vi "SVT UFF58 Write Spectrum (Complex) (N Ch).vi"(0 "file refnum":refnum<k20>, 1 "ID lines (1-3)":T8[](array[typedef]), 2 "data precision (double-precision:1)":T1=1 items=["single-precision", "double-precision"], 5 "real part":cluster{"x0":dbl, "dx":dbl, "Y Real":dbl[]}[](array[cluster]) {"Y Real" format="%.2f"; "dx" format="%.2f"; "x0" format="%.2f"}, 7 "imaginary part":cluster{"x0":dbl, "dx":dbl, "Y Im":dbl[]}[](array[cluster]) {"Y Im" format="%.2f"; "dx" format="%.2f"; "x0" format="%.2f"}, 9 "spectrum info":T2[](array[typedef]) {"x-axis units" items=["Time (s)"=0, "Frequency-CB (Hz)"=1, "Frequency-CPB (Hz)"=1248, "Frequency-Arbitrary (Hz)"=2357, "Quefrency (s)"=2, "Revolutions (rev)"=3, "Order"=4, "Speed (RPM)"=11, "Speed (rad/s)"=21, "Index"=65535]; "weighting filter" items=["Linear", "A-weighting", "B-weighting", "C-weighting", "ITU-R 468-4", "Dolby", "CCITT", "C-message", "Wb", "Wc", "Wd", "We", "Wf", "Wh", "Wj", "Wk", "Wm", "AES17 20 kHz lowpass", "AES17 40 kHz lowpass", "AES17 20 kHz highpass", "AES17 40 kHz highpass"]; "dB reference [EU]" format="%.2f"; "engineering units" items=["custom..."=0, "V"=1, "A"=21, "C"=30, "pC"=31, "s"=32, "-"=29, "Pa"=2, "N"=20, "g"=3, "m/s^2"=4, "m/s"=5, "m"=6, "mm/s"=12, "mm"=13, "micron/s"=14, "micron"=15, "in/s^2"=7, "in/s"=8, "in"=9, "mil/s"=10, "mil"=11, "rad/s^2"=16, "rad/s"=17, "rad"=18, "deg/s^2"=26, "deg/s"=27, "deg"=28, "RPM"=22, "cycle/s^2"=23, "Hz"=24, "cycle"=25, "strain"=19]; "spectral info"."window" items=["None "=0, "Hanning"=1, "Hamming"=2, "Blackman-Harris"=3, "Exact Blackman"=4, "Blackman"=5, "Flat Top"=6, "4 Term B-Harris "=7, "7 Term B-Harris"=8, "Low Sidelobe"=9, "Force - Exponential"=10, "Gaussian"=62]}, 11 "error in (no error)":errorcluster) -> (4 "dup file refnum":refnum<k20>, 6 "function refnums":refnum<k20>[](array[refnum]), 15 "error out":errorcluster)   [LabVIEW 2017, in "SoundVib_UFF58.lvlib"]
doc: "Writes data to the UFF58 (universal file format) file specified by the <B>file refnum</B> input. This VI also writes the fields in records 1, 2, and 3, <B>ID lines (1-3)</B>. You can write a single time domain waveform, multiple time domain waveforms, a single real frequency spectrum, multiple real frequency spectra, a single complex frequency spectrum, multiple complex frequency spectra, or generic data to a UFF file. If a frequency spectrum is in decibels, this VI converts the spectrum to linear before writing to the UFF58 file. The default instance, SVT UFF58 Write Time Waveform (1 Ch), writes a single time domain waveform to the file specified by the <B>file refnum</B> input. Wire data to the <B>file refnum</B> input to determine the polymorphic instance to use or manually select the instance."
uses:
  <vilib>/addons/Sound and Vibration/svt_UFF58/SoundVib_UFF58.lvlib
  <vilib>/addons/Sound and Vibration/svt_UFF58/subVIs/sv_IDLines123.ctl
  <vilib>/addons/_NISVFA/_Shared subVIs/Controls/svc_Spectrum Info.ctl
  <vilib>/addons/_NISVFA/_Shared subVIs/Controls/svc_X-Axis Units.ctl
  <vilib>/addons/_NISVFA/_Shared subVIs/Controls/svc_Spectrum Type.ctl
  <vilib>/addons/_NISVFA/_Shared subVIs/Controls/svc_Engineering Units Text Ring.ctl
  <vilib>/addons/_NISVFA/_Shared subVIs/Controls/svc_Weighting Filter Text Ring.ctl
  <vilib>/addons/_NISVFA/_Shared subVIs/Controls/svc_Complimentary Spectrum Units.ctl
  <vilib>/addons/Sound and Vibration/svt_UFF58/subVIs/sv_UFF58 Data Precision.ctl
  <vilib>/addons/Sound and Vibration/svt_UFF58/subVIs/sv_UFF58 Check Data Valid (Freq - Complex) (N Ch).vi
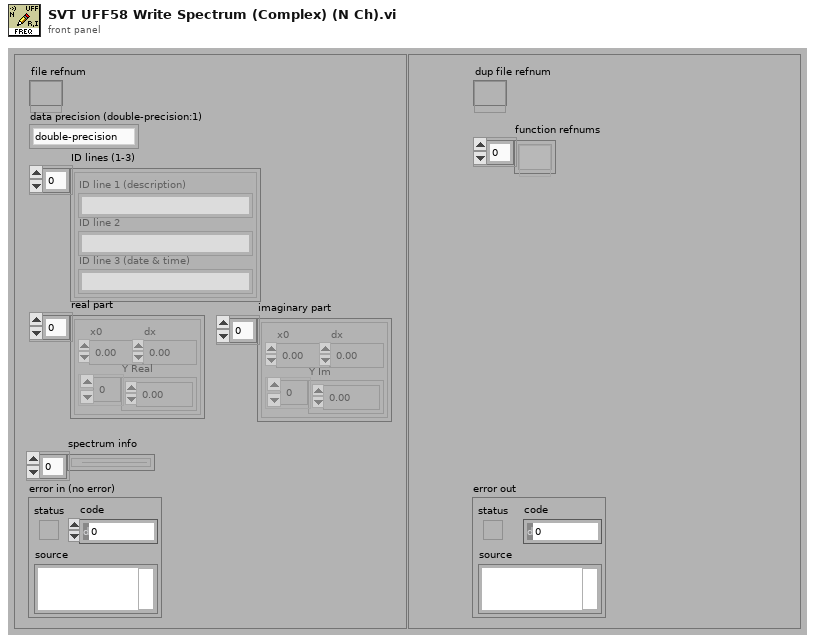
[diagram p1: front panel]
types:
  T1 = typedef "SoundVib_UFF58.lvlib/sv_UFF58 Data Precision.ctl" = u32
  T2 = typedef "svc_Spectrum Info.ctl" = cluster{"channel name":string, "description":string, "x-axis units":T3, "spectral info":cluster{"spectrum type":T4, "linear/dB":enum16{"linear", "dB"}, "window":u16, "window size":i32, "FFT size":i32}, "engineering units":T5, "custom label":string, "dB reference [EU]":dbl, "peak units":enum16{"rms", "peak", "peak-peak"}, "weighting filter":T6, "spectral density?":bool, "unit label":string, "spectrum skewed?":bool, "complimentary spectrum units":T7}
  T3 = typedef "svc_X-Axis Units.ctl" = u16
  T4 = typedef "svc_Spectrum Type.ctl" = enum16{"FFT Spectrum [complex]", "Amplitude [Magnitude]", "Power [Magnitude^2]", "Cross Spectrum [complex]", "Frequency Response [Complex]"}
  T5 = typedef "svc_Engineering Units Text Ring.ctl" = u16
  T6 = typedef "svc_Weighting Filter Text Ring.ctl" = u16
  T7 = typedef "svc_Complimentary Spectrum Units.ctl" = enum16{"none", "radians", "degrees", "cycles", "imaginary"}
  T8 = typedef "SoundVib_UFF58.lvlib/sv_IDLines123.ctl" = cluster{"ID line 1 (description)":string, "ID line 2":string, "ID line 3 (date & time)":string}
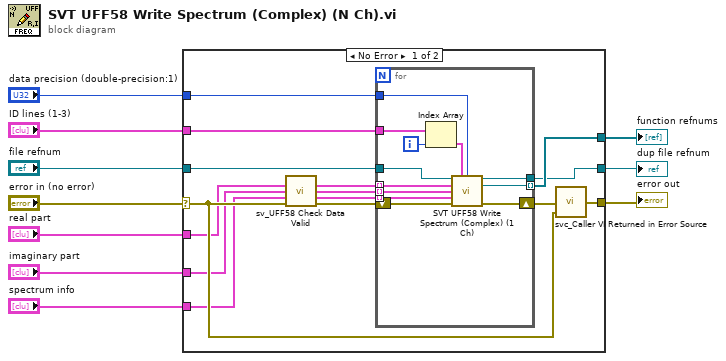
[diagram p0: block diagram]
diagram:
  n1 = case shown="No Error" "error in (no error)" {
    selector: "error in (no error)" -> [w17 w39]
    tunnel: "file refnum" -> [w25 w38]
    tunnel: "spectrum info" -> [w12 _]
    tunnel: "ID lines (1-3)" -> [w14 _]
    tunnel: [w24 _] -> w7
    tunnel: "real part" -> [w16 _]
    tunnel: "imaginary part" -> [w15 _]
    tunnel: [w18 w39] -> w4
    tunnel: [w23 w38] -> w3
    tunnel: "data precision (double-precision:1)" -> [w13 _]
    frame No Error {
      n2 = call-poly <vilib>:"sv_UFF58 Check Data Valid.vi"("real part in"=w16, "imaginary part in"=w15, "spectrum info in"=w12, "error in (no error)"=w17) -> ("real part out"=w21:cluster{"f0":dbl, "df":dbl, "magnitude":dbl[]}[], "imaginary part out"=w20:cluster{"f0":dbl, "df":dbl, "magnitude":dbl[]}[], "spectrum info out"=w11:T2[], "error out"=w22:errorcluster)  [unwired: 8 in]
      n3 = for {
        tunnel: w25 -> [w37]
        shift-right: [w34] -> w19
        shift-left: w22 -> [w36]
        tunnel: w11 -> [w32] mode=indexing
        tunnel: w14 -> [w31]
        tunnel: [w35] -> w23
        tunnel: [w33] -> w24 mode=indexing
        tunnel: w21 -> [w29] mode=indexing
        tunnel: w20 -> [w28] mode=indexing
        tunnel: w13 -> [w26]
        i -> [w30]
        n4 = Index Array(array=w31, index=w30) -> (element=w27:T8)
        n5 = call <vilib>:"SVT UFF58 Write Spectrum (Complex) (1 Ch).vi"("file refnum"=w37, "ID lines (1-3)"=w27, "data precision (double-precision:1)"=w26, "real part"=w29, "imaginary part"=w28, "spectrum info"=w32, "error in (no error)"=w36) -> ("dup file refnum"=w35:refnum<k20>, "function refnum"=w33:refnum<k20>, "error out"=w34:errorcluster)  [unwired: 6 in]
      }
      n6 = call <vilib>:"svc_Caller VI Returned in Error Source.vi"("warning input to caller"=w17, "error in (no error)"=w19) -> ("error out"=w18:errorcluster)  [unwired: 3 in]
    }
    frame Error {
    }
  }
  "function refnums" <- w7
  "dup file refnum" <- w3
  "error out" <- w4
